vi "Test Serialize Signed Integers.vi"(8 "error in (no error)":errorcluster) -> (0 "error out":errorcluster)   [LabVIEW 2013]
uses:
  src/Serializer/JSON Serializer/JSON Serializer.lvclass
  <vilib>/addons/_JKI Toolkits/Caraya/classes/Test/Test.lvclass
  <vilib>/addons/_JKI Toolkits/Caraya/classes/Assert/Assert.lvclass
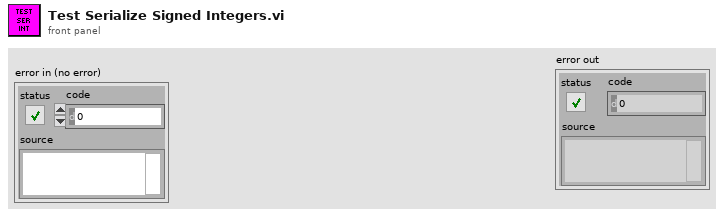
[diagram p1: front panel]
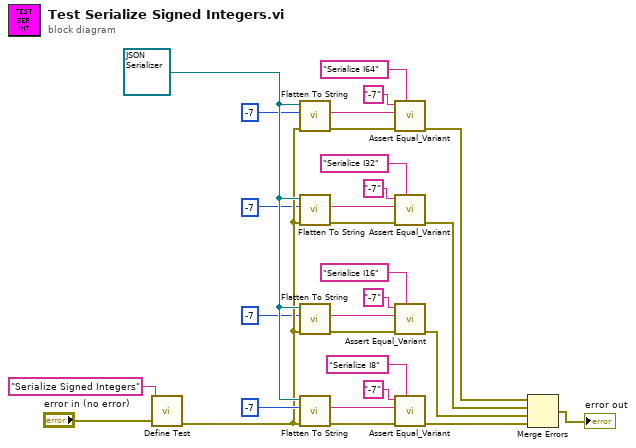
[diagram p0: block diagram]
diagram:
  w11 = refnum<class "JSON Serializer.lvclass"> refnum ("JKI JSON Serialization.lvlib:JSON Serializer.lvclass")
  n1 = call <vilib>:"Define Test.vi"("error in (no error)"="error in (no error)", "Label (VI Title)"="Serialize Signed Integers") -> ("error out"=w10:errorcluster)  [unwired: 9 in]
  n2 = call-dynamic "Flatten To String.vi"("error in (no error)"=w10, "Variant"=i64 -7, "JSON Serializer in"=w11) -> ("error out"=w15:errorcluster, "String"=w14:string)  [unwired: 6 in, 1 out]
  n3 = call-dynamic "Flatten To String.vi"("error in (no error)"=w10, "Variant"=-7, "JSON Serializer in"=w11) -> ("error out"=w19:errorcluster, "String"=w18:string)  [unwired: 6 in, 1 out]
  n4 = call-dynamic "Flatten To String.vi"("error in (no error)"=w10, "Variant"=i16 -7, "JSON Serializer in"=w11) -> ("error out"=w23:errorcluster, "String"=w22:string)  [unwired: 6 in, 1 out]
  n5 = call-dynamic "Flatten To String.vi"("error in (no error)"=w10, "Variant"=i8 -7, "JSON Serializer in"=w11) -> ("error out"=w27:errorcluster, "String"=w26:string)  [unwired: 6 in, 1 out]
  n6 = call <vilib>:"Assert Equal_Variant.vi"("Label"="Serialize I64", "error in (no error)"=w15, "Y"=w14, "X"="-7") -> ("error out"=w5:errorcluster)  [unwired: 7 in]
  n7 = call <vilib>:"Assert Equal_Variant.vi"("Label"="Serialize I32", "error in (no error)"=w19, "Y"=w18, "X"="-7") -> ("error out"=w6:errorcluster)  [unwired: 7 in]
  n8 = call <vilib>:"Assert Equal_Variant.vi"("Label"="Serialize I16", "error in (no error)"=w23, "Y"=w22, "X"="-7") -> ("error out"=w7:errorcluster)  [unwired: 7 in]
  n9 = call <vilib>:"Assert Equal_Variant.vi"("Label"="Serialize I8", "error in (no error)"=w27, "Y"=w26, "X"="-7") -> ("error out"=w8:errorcluster)  [unwired: 7 in]
  n10 = Merge Errors(w5, w6, w7, w8) -> (→"error out":errorcluster)
